vi "Wheel Check.vi"(8 "Trigger 2":bool, 9 "Trigger 1":bool, 10 "Right Drive":dbl, 11 "Left Drive":dbl) -> (1 "Right Out":dbl, 2 "Left Out":dbl)   [LabVIEW 2011]
uses:
  Robot Global Data.vi
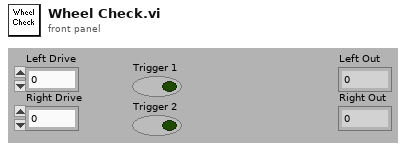
[diagram p1: front panel]
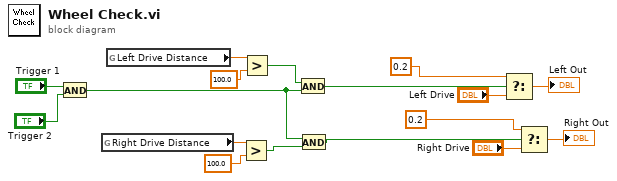
[diagram p0: block diagram]
diagram:
  n1 = And(x="Trigger 1", y="Trigger 2") -> (x .and. y?=w8:bool)
  n2 = global read "Robot Global Data.vi" "Right Drive Distance"() -> (w11:dbl)
  n3 = global read "Robot Global Data.vi" "Left Drive Distance"() -> (w9:dbl)
  n4 = Greater?(x=w11, y=100.0) -> (0:w13:bool)
  n5 = Greater?(x=w9, y=100.0) -> (0:w12:bool)
  n6 = And(x=w12, y=w8) -> (x .and. y?=w14:bool)
  n7 = And(x=w8, y=w13) -> (x .and. y?=w17:bool)
  n8 = Select(t=0.2, s=w14, f="Left Drive") -> (s? t:f=→"Left Out":dbl)
  n9 = Select(t=0.2, s=w17, f="Right Drive") -> (s? t:f=→"Right Out":dbl)
